vi "Find Keywords.vi"(7 "searched objects":string[](array[string]), 8 "error in (no error)":errorcluster, 10 "attributes":string[](array[string]), 11 "errors":T2[](array[typedef])) -> (0 "error out":errorcluster, 3 "filtered IDs":T1[](array[typedef]))   [LabVIEW 2017]
uses:
  Error File Management/Controls/NI Error.ctl
  Error List/Error Owner and ID.ctl
  <vilib>/regexp/Match Regular Expression.xnode
  Error File Management/Error File Management.lvlib
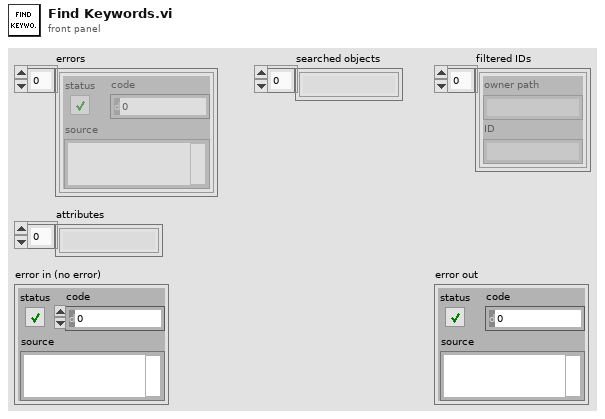
[diagram p1: front panel]
types:
  T1 = typedef "Error Owner and ID.ctl" = cluster{"owner path":string, "ID":string}
  T2 = typedef "Error File Management.lvlib/NI Error.ctl" = errorcluster
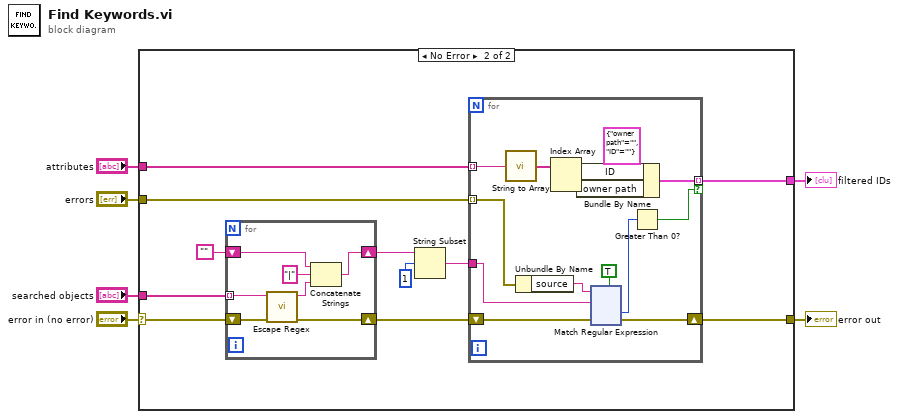
[diagram p0: block diagram]
diagram:
  n1 = case shown="No Error" "error in (no error)" {
    selector: "error in (no error)" -> [w7 w14]
    tunnel: "searched objects" -> [_ w16]
    tunnel: [w7 w15] -> w4
    tunnel: "errors" -> [_ w10]
    tunnel: "attributes" -> [_ w9]
    tunnel: [_ w8] -> w1
    frame Error {
    }
    frame No Error {
      n2 = for {
        tunnel: w16 -> [w153] mode=indexing
        shift-right: [w149] -> w13
        shift-left: "" -> [w152]
        shift-right: [w148] -> w18
        shift-left: w14 -> [w147]
        n3 = call "Escape Regex.vi"("error in (no error)"=w147, "regex"=w153) -> ("error out"=w148:errorcluster, "escaped regex"=w151:string)  [unwired: 8 in]
        n4 = Concatenate Strings(w152, "|" ("string"), w151) -> (w149:string)
      }
      n5 = String Subset(string=w13, offset (0)=1) -> (substring=w11:string)  [unwired: 1 in]
      n6 = for {
        tunnel: w11 -> [w31]
        shift-right: [w27] -> w15
        shift-left: w18 -> [w29]
        tunnel: w10 -> [w26] mode=indexing
        tunnel: w9 -> [w22] mode=indexing
        tunnel: [w20] -> w8 mode=indexing if=w19
        n7 = call "String to Array.vi"("string"=w22) -> ("array"=w25:string[])  [unwired: 1 in]
        n8 = Unbundle By Name(w26) -> ("source"=w32:string)
        n9 = Index Array(array=w25) -> (element #1=w24:string, element #2=w23:string)  [unwired: 2 in]
        n10 = Bundle By Name(cluster=T1 {"owner path"="", "ID"=""} ("owner error"), "ID"=w24, "owner path"=w23) -> (w20:T1)
        n11 = xnode "Match Regular Expression"("input string"=w32, "regular expression"=w31, "error in"=w29, "multiline? (F)"=TRUE) -> ("offset past match"=w28:i32, "error out"=w27:errorcluster)  [unwired: 2 in, 3 out]
        n12 = Greater Than 0?(x=w28) -> (x > 0?=w19:bool)
      }
    }
  }
  "error out" <- w4
  "filtered IDs" <- w1
